vi "ApplyLayoutToObject.vi"(5 "scaling settings":T1={"scaling factor"={"horizontal"=1.0, "vertical"=1.0}, "scaling to ignore"=variant} {"scaling factor"."vertical" min=0.0; "scaling factor"."horizontal" min=0.0}, 7 "properties to ignore":variant, 8 "error in (no error)":errorcluster, 10 "GObj Refnum":refnum<vi>, 11 "Ring Layout in":refnum<class "Ring Layout.lvclass">) -> (0 "error out":errorcluster, 3 "Ring Layout out":refnum<class "Ring Layout.lvclass">)   [LabVIEW 2010, in "NI_SE_Front Panel Layout.lvlib" / "Ring Layout.lvclass"]
doc: "Apply layout information to the GObj Refnum."
uses:
  Ring Layout.lvclass
  Scaling Factor_Options.ctl
  XY Scaling Factor.ctl
  NamedNumeric Control Layout/NamedNumeric Control Layout.lvclass
  Ring Layout.lvclass/Ring Layout.ctl
  Properties To Ignore.vi
  NI_SE_Front Panel Layout.lvlib
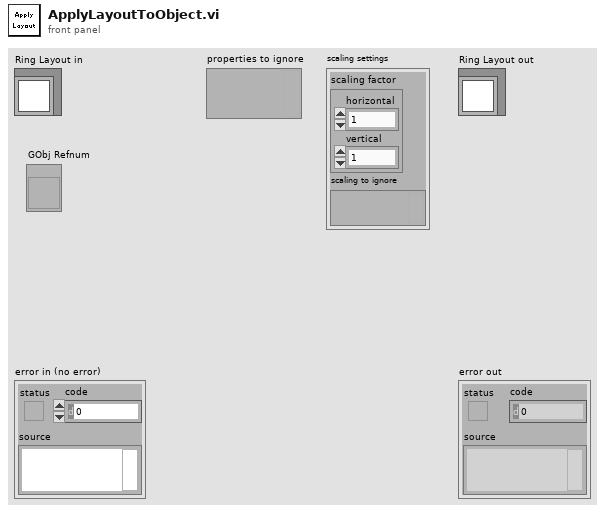
[diagram p1: front panel]
types:
  T1 = typedef "NI_SE_Front Panel Layout.lvlib/Scaling Factor_Options.ctl" = cluster{"scaling factor":T2, "scaling to ignore":variant}
  T2 = typedef "NI_SE_Front Panel Layout.lvlib/XY Scaling Factor.ctl" = cluster{"horizontal":dbl, "vertical":dbl}
  T3 = enum32{"Text Ring", "Pict Ring", "Text and Pict Ring"}
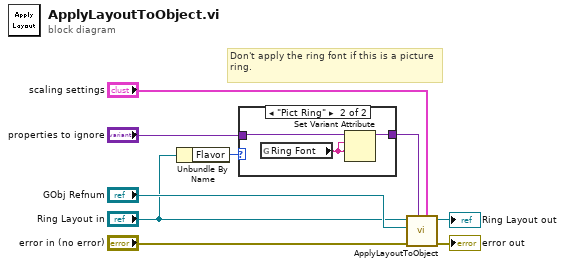
[diagram p0: block diagram]
diagram:
  # "Don't apply the ring font if this is a picture ring."
  n1 = Unbundle By Name("Ring Layout in") -> ("Flavor"=w3:T3)
  n2 = case shown="\"Pict Ring\"" w3 {
    tunnel: "properties to ignore" -> [w10 w13]
    tunnel: [w10 w12] -> w1
    frame Default {
    }
    frame "Pict Ring" {
      n3 = global read "Properties To Ignore.vi" "Ring Font"() -> (w11:string)
      n4 = Set Variant Attribute(Variant=w13, name=w11, value=w11) -> (Variant out=w12:variant)  [unwired: 1 in, 2 out]
    }
  }
  n5 = call-parent "ApplyLayoutToObject.vi"("scaling settings"="scaling settings", "properties to ignore"=w1, "error in (no error)"="error in (no error)", "GObj Refnum"="GObj Refnum", "NamedNumeric Control Layout in"="Ring Layout in") -> ("error out"=→"error out":errorcluster, "NamedNumeric Control Layout out"=→"Ring Layout out":refnum<class "Ring Layout.lvclass">)  [unwired: 5 in]
